vi "dfd_Normalized Lattice to Lattice.vi"(11 "k & ^k":dbl[](array[numeric]) format="%.2f") -> (2 "^k [M~1]":dbl[](array[numeric]) format="%.2f", 3 "k [M~1]":dbl[](array[numeric]) format="%.2f")   [LabVIEW 2017, in "NI_DigFilterLicensed.lvlib"]
uses:
  <vilib>/addons/Digital Filter Design/NI_DigFilterLicensed.lvlib
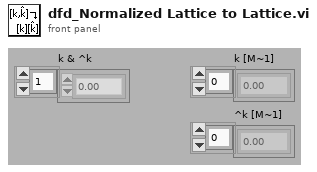
[diagram p1: front panel]
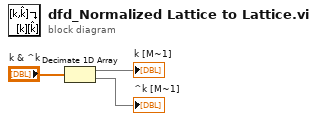
[diagram p0: block diagram]
diagram:
  n1 = Decimate 1D Array("k & ^k") -> (→"k [M~1]":dbl[], →"^k [M~1]":dbl[])
